vi "Get_TSL_APC_Max_MinPower.vi"(8 "error in (no error)":errorcluster, 9 "Counter_570":i32, 10 "数组":T1(array[cluster]), 11 "TSL":refnum<k24>[](array[refnum])) -> (0 "error out":errorcluster, 1 "TSL out":refnum<k24>[](array[refnum]), 2 "minpower":dbl=-9999.0, 3 "maxpower":dbl=9999.0)   [LabVIEW 2017]
doc: "get the APC max/min power for TSL"
uses:
  LV_IL_Sample/DLL/InstrumentDLL.dll
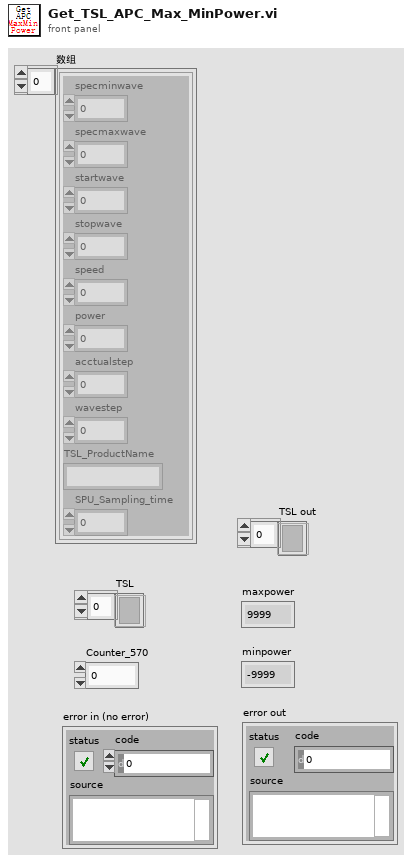
[diagram p1: front panel]
types:
  T1 = cluster{"specminwave":dbl, "specmaxwave":dbl, "startwave":dbl, "stopwave":dbl, "speed":dbl, "power":dbl, "acctualstep":dbl, "wavestep":dbl, "TSL_ProductName":string, "SPU_Sampling_time":dbl}[]
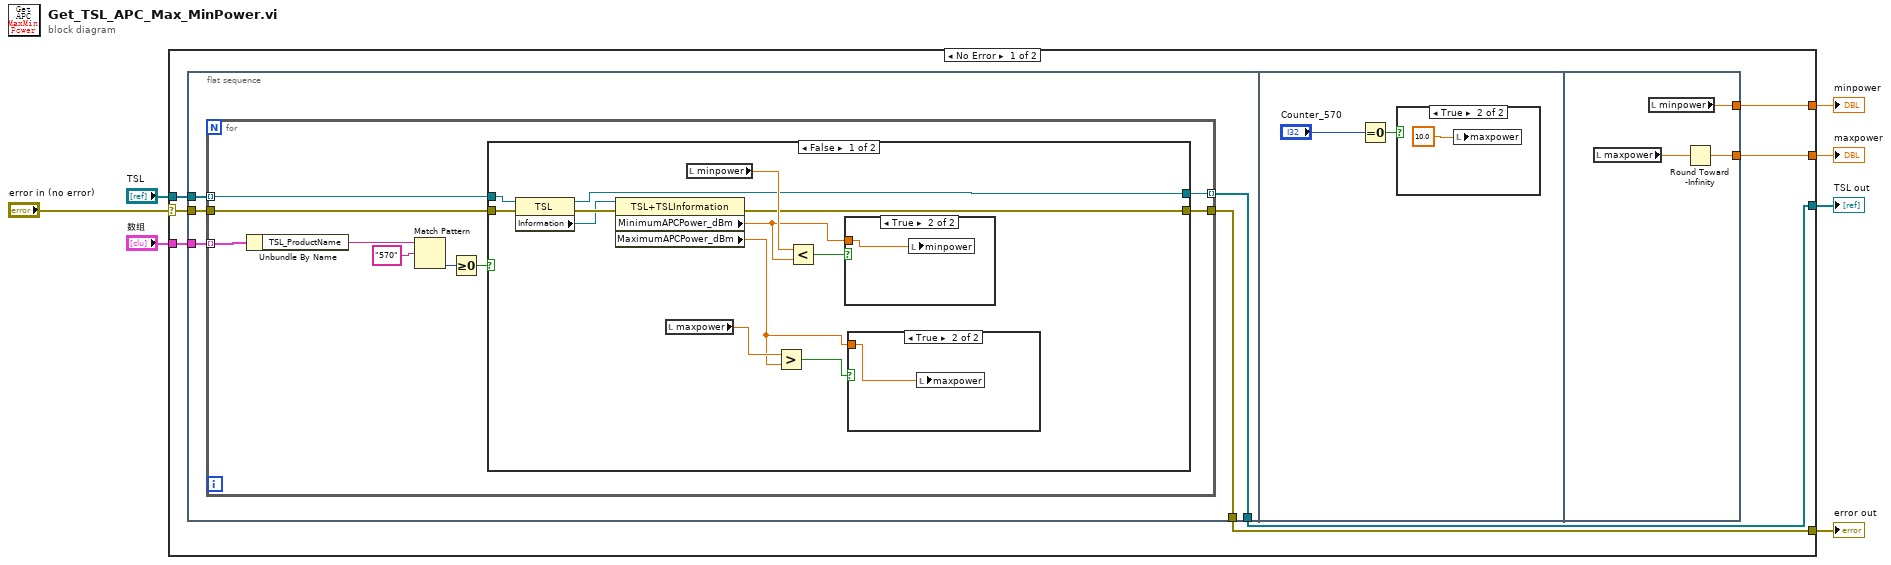
[diagram p0: block diagram]
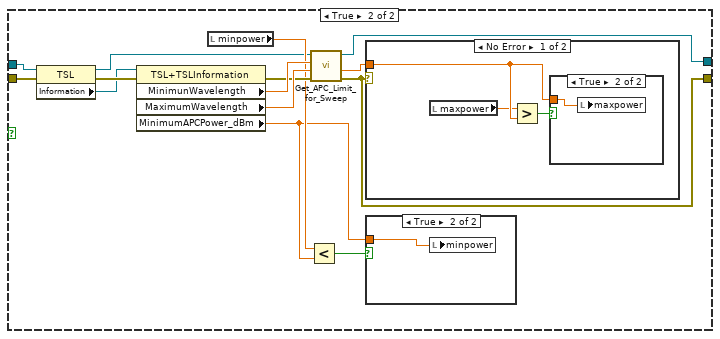
[diagram p4: hidden frame]
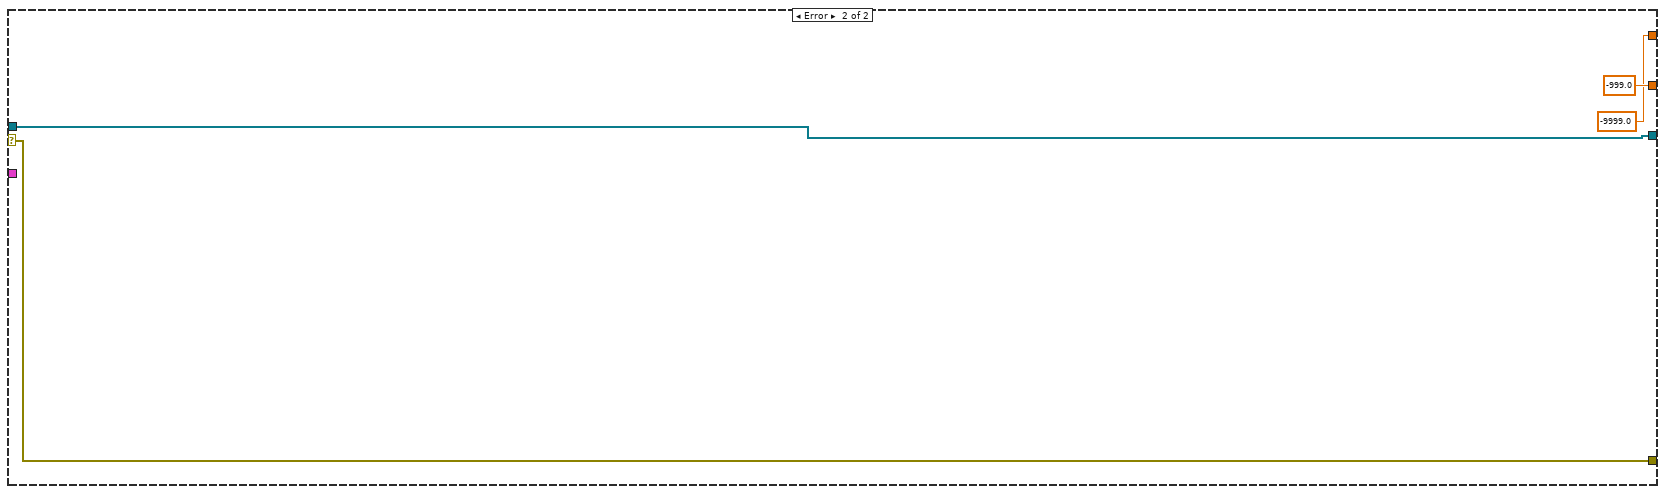
[diagram p9: hidden frame]
diagram:
  n1 = case shown="No Error" "error in (no error)" {
    selector: "error in (no error)" -> [w11 w71]
    tunnel: [w14 -999.0] -> w7
    tunnel: "数组" -> [w13 _]
    tunnel: "TSL" -> [w12 w68]
    tunnel: [w10 w71] -> w3
    tunnel: [w9 -9999.0 ("minpower")] -> w2
    tunnel: [w8 w68] -> w1
    frame No Error {
      n2 = flat-sequence {
        tunnel: w12 -> [w19]
        tunnel: w13 -> [w18]
        tunnel: w11 -> [w17]
        tunnel: [w16] -> w10
        tunnel: [w15] -> w8
        tunnel: [w67] -> w14
        tunnel: [w65] -> w9
        frame #0 {
          n3 = for {
            tunnel: w19 -> [w23] mode=indexing
            tunnel: w18 -> [w26] mode=indexing
            tunnel: w17 -> [w22]
            tunnel: [w21] -> w16
            tunnel: [w20] -> w15 mode=indexing
            n4 = Unbundle By Name(w26) -> ("TSL_ProductName"=w28:string)
            n5 = Match Pattern(string=w28, regular expression="570" ("正则表达式")) -> (offset past match=w25:i32)  [unwired: 1 in, 3 out]
            n6 = Greater Or Equal To 0?(x=w25) -> (x >= 0?=w24:bool)
            n7 = case shown="False" w24 {
              tunnel: w23 -> [w38 w44]
              tunnel: w22 -> [w37 w50]
              tunnel: [w33 w49] -> w21
              tunnel: [w32 w45] -> w20
              frame False {
                n8 = property on="属性节点" class="TSL"(reference=w38, error in=w37) -> (reference out=w32:refnum<k24>, error out=w40:errorcluster, "Information"=w39:refnum<k24>)
                n9 = property on="属性节点" class="TSL+TSLInformation"(reference=w39, error in=w40) -> (error out=w33:errorcluster, "MinimumAPCPower_dBm"=w34:dbl, "MaximumAPCPower_dBm"=w29:dbl)  [unwired: 1 out]
                n10 = local read "maxpower"() -> (w30:dbl)
                n11 = local read "minpower"() -> (w36:dbl)
                n12 = Greater?(x=w30, y=w29) -> (0:w31:bool)
                n13 = Less?(x=w36, y=w34) -> (x < y?=w35:bool)
                n14 = case shown="True" w35 {
                  tunnel: w34 -> [_ w42]
                  frame False {
                  }
                  frame True {
                    n15 = local write "minpower"(w42) -> ()
                  }
                }
                n16 = case shown="True" w31 {
                  tunnel: w29 -> [_ w41]
                  frame False {
                  }
                  frame True {
                    n17 = local write "maxpower"(w41) -> ()
                  }
                }
              }
              frame True {
                n18 = property on="属性节点" class="TSL"(reference=w44, error in=w50) -> (reference out=w43:refnum<k24>, error out=w56:errorcluster, "Information"=w55:refnum<k24>)
                n19 = property on="属性节点" class="TSL+TSLInformation"(reference=w55, error in=w56) -> (error out=w52:errorcluster, "MinimunWavelength"=w54:dbl, "MaximumWavelength"=w53:dbl, "MinimumAPCPower_dBm"=w46:dbl)  [unwired: 1 out]
                n20 = local read "minpower"() -> (w48:dbl)
                n21 = Less?(x=w48, y=w46) -> (x < y?=w47:bool)
                n22 = call "Get_APC_Limit_for_Sweep.vi"("error in (no error)"=w52, "maxwave"=w53, "minwave"=w54, ".NET Reference in"=w43) -> ("error out"=w49:errorcluster, "maxpower"=w51:sgl, "Reference out"=w45:refnum<k24>)  [unwired: 5 in]
                n23 = case shown="No Error" w49 {
                  tunnel: w51 -> [w59 _]
                  frame No Error {
                    n24 = local read "maxpower"() -> (w58:dbl)
                    n25 = Greater?(x=w58, y=w59) -> (0:w60:bool)
                    n26 = case shown="True" w60 {
                      tunnel: w59 -> [_ w61]
                      frame False {
                      }
                      frame True {
                        n27 = local write "maxpower"(w61) -> ()
                      }
                    }
                  }
                  frame Error {
                  }
                }
                n28 = case shown="True" w47 {
                  tunnel: w46 -> [_ w57]
                  frame False {
                  }
                  frame True {
                    n29 = local write "minpower"(w57) -> ()
                  }
                }
              }
            }
          }
        }
        frame #1 {
          n30 = Equal To 0?(x="Counter_570") -> (x = 0?=w63:bool)
          n31 = case shown="True" w63 {
            frame False {
            }
            frame True {
              n32 = local write "maxpower"(10.0 ("maxpower")) -> ()
            }
          }
        }
        frame #2 {
          n33 = local read "maxpower"() -> (w66:dbl)
          n34 = local read "minpower"() -> (w65:dbl)
          n35 = Round Toward -Infinity(1:w66) -> (0:w67:dbl)
        }
      }
    }
    frame Error {
    }
  }
  "maxpower" <- w7
  "error out" <- w3
  "minpower" <- w2
  "TSL out" <- w1
